vi "HMI Main.vi"() -> ()   [LabVIEW 2014]
panel:
  out "Connected?":bool
  in  "PID Parameters":cluster{"Kp":dbl, "Ki":dbl, "Kd":dbl}
  in  "Set Points":dbl(slide) scale=-10.0..10.0
  in  "RT Target IP":string
  in  "Updata Parameters":bool
  in  "Stop Control":bool
  in  "Start Control":bool
  in  "Connect to Target":bool
  in  "Exit":bool
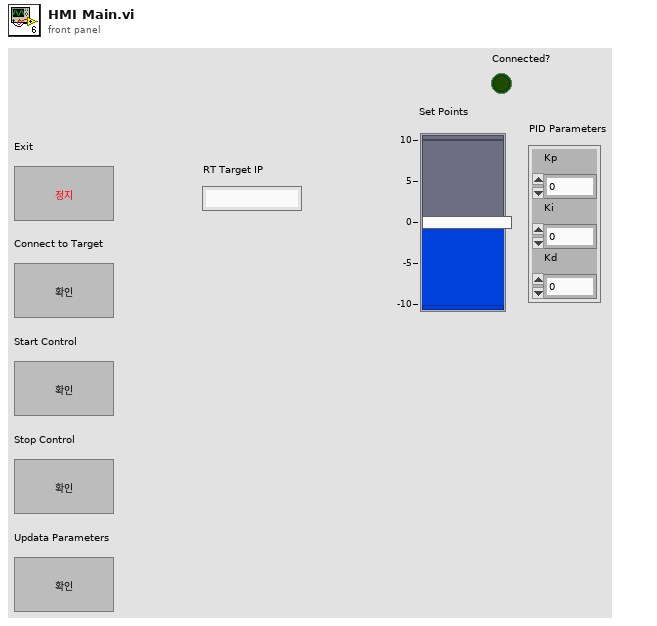
[diagram p1: front panel]
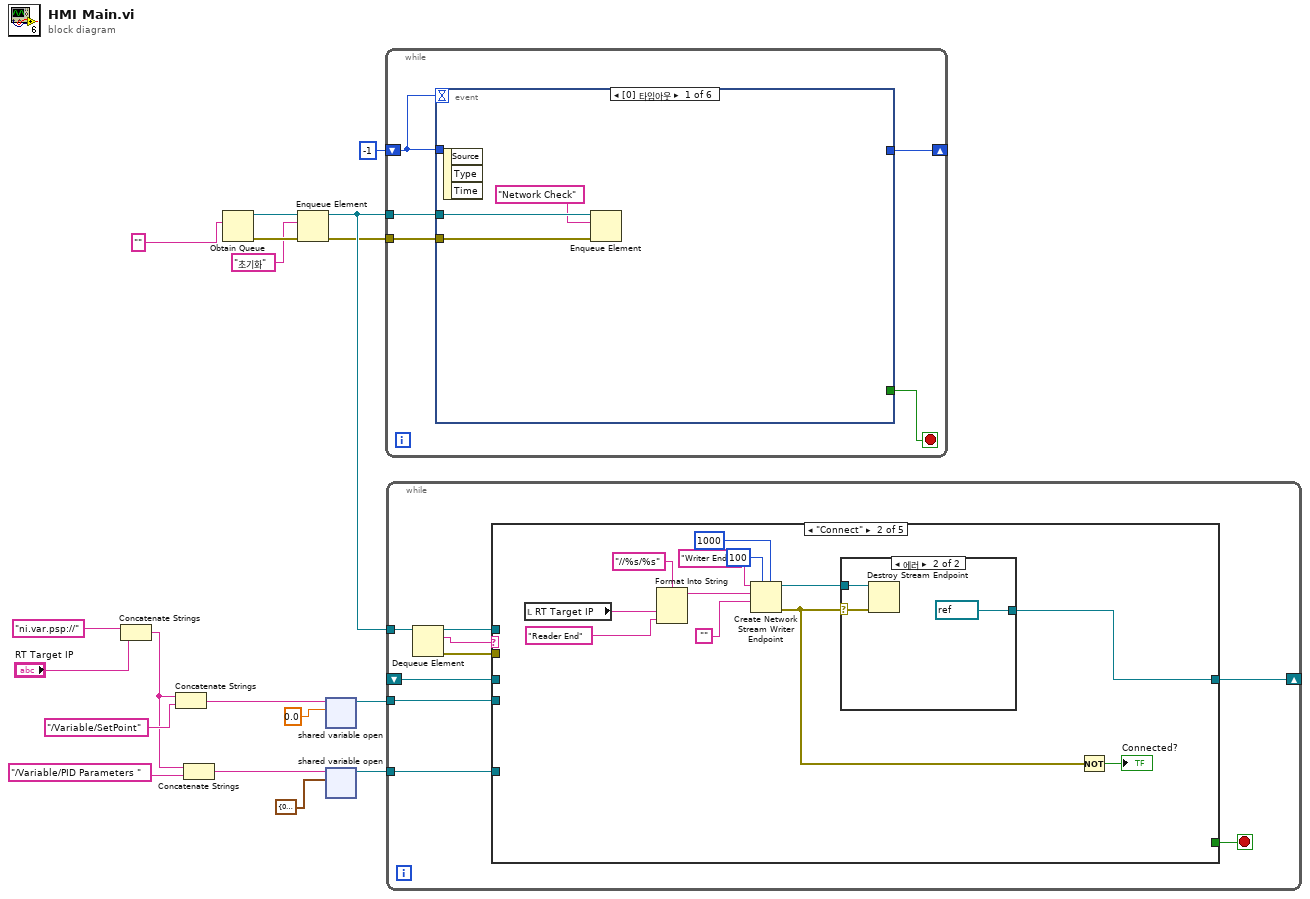
[diagram p0: block diagram]
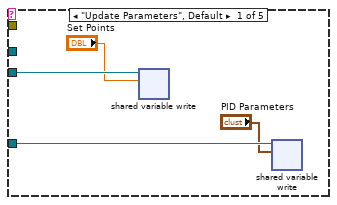
[diagram p2: hidden frame]
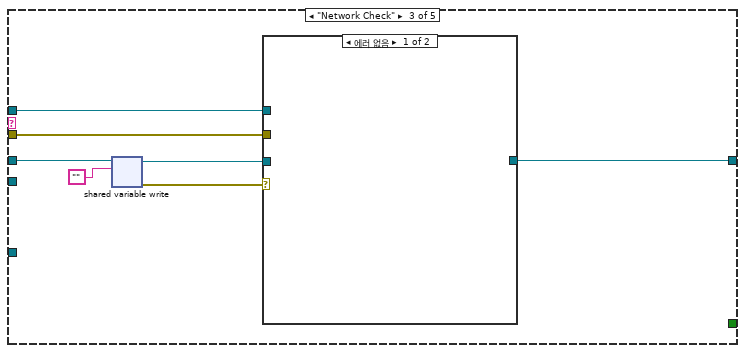
[diagram p4: hidden frame]
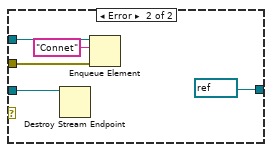
[diagram p5: hidden frame]
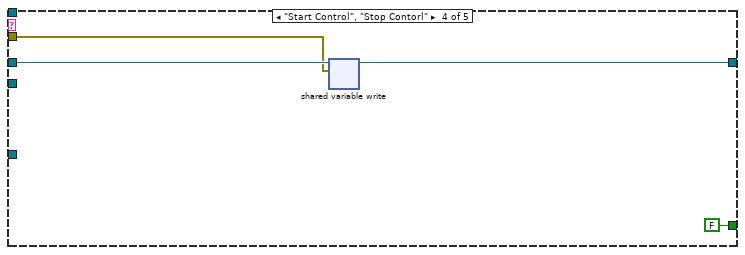
[diagram p6: hidden frame]
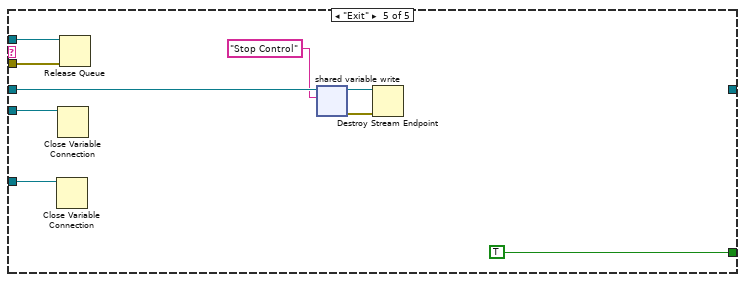
[diagram p7: hidden frame]
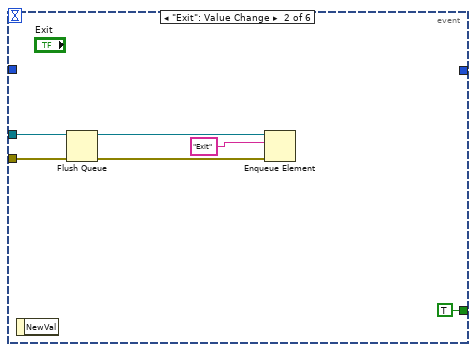
[diagram p8: hidden frame]
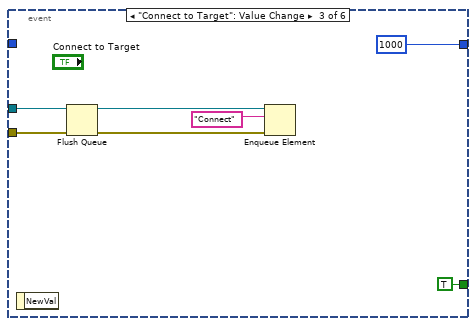
[diagram p9: hidden frame]
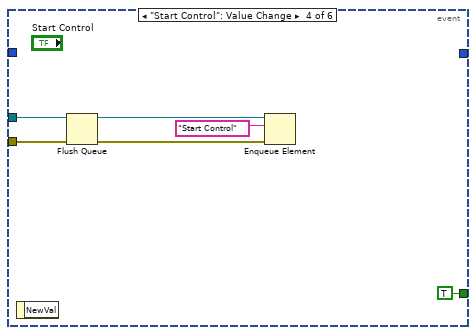
[diagram p10: hidden frame]
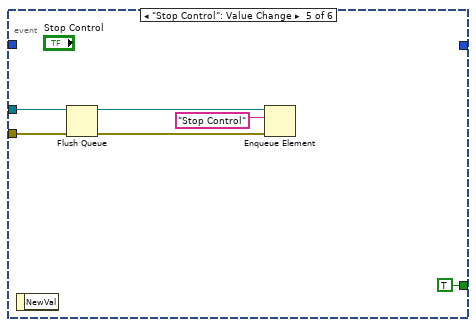
[diagram p11: hidden frame]
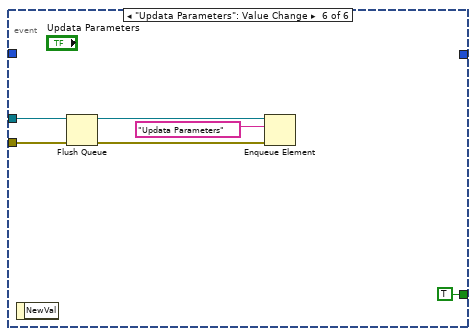
[diagram p12: hidden frame]
diagram:
  n1 = Concatenate Strings("ni.var.psp://", "RT Target IP") -> (w8:string)
  n2 = Concatenate Strings(w8, "/Variable/SetPoint") -> (w6:string)
  n3 = Concatenate Strings(w8, "/Variable/PID Parameters ") -> (w4:string)
  n4 = Obtain Queue(element data type="") -> (queue out=w16:refnum<queue>, error out=w17:errorcluster)  [unwired: 4 in, 1 out]
  n5 = Enqueue Element(queue=w16, element="초기화" ("원소"), error in (no error)=w17) -> (queue out=w15:refnum<queue>, error out=w13:errorcluster)  [unwired: 1 in, 1 out]
  n6 = shared-variable-open(w6, 0.0) -> (w7:refnum<k21>)  [unwired: 2 in, 1 out]
  n7 = shared-variable-open(w4, cluster{"Kp":dbl, "Ki":dbl, "Kd":dbl} {"Kp"=0.0, "Ki"=0.0, "Kd"=0.0} ("PID Parameters")) -> (w5:refnum<k21>)  [unwired: 2 in, 1 out]
  n8 = while {
    tunnel: w15 -> [w23]
    tunnel: w13 -> [w22]
    shift-right: [w20] -> _
    shift-left: -1 -> [w19]
    stop <- w21 stop-if-true
    n9 = event shown="[0] 타임아웃" {
      selector: _ -> [_ _ _ _ _ _]
      dyn-events: _ -> [_ _ _ _ _ _]
      timeout: w19 -> [_ _ _ _ _ _]
      tunnel: w23 -> [w26 w32 w39 w45 w51 w57]
      tunnel: w22 -> [w25 w31 w38 w44 w50 w56]
      tunnel: [_ TRUE TRUE TRUE TRUE TRUE] -> w21
      tunnel: [_ _ 1000 _ _ _] -> w20
      tunnel: w19 -> [_ _ _ _ _ _]
      event Timeout {
        n10 = event-data() -> ()  [unwired: 1 in, 3 out]
        n11 = Enqueue Element(queue=w26, element="Network Check" ("원소"), error in (no error)=w25) -> ()  [unwired: 1 in, 3 out]
      }
      event "Exit": Value Change {
        n12 = event-data() -> ()  [unwired: 1 in, 1 out]
        n13 = Flush Queue(queue=w32, error in (no error)=w31) -> (queue out=w29:refnum<queue>, error out=w28:errorcluster)  [unwired: 1 out]
        n14 = Enqueue Element(queue=w29, element="Exit", error in (no error)=w28) -> ()  [unwired: 1 in, 3 out]
      }
      event "Connect to Target": Value Change {
        n15 = event-data() -> ()  [unwired: 1 in, 1 out]
        n16 = Flush Queue(queue=w39, error in (no error)=w38) -> (queue out=w36:refnum<queue>, error out=w35:errorcluster)  [unwired: 1 out]
        n17 = Enqueue Element(queue=w36, element="Connect", error in (no error)=w35) -> ()  [unwired: 1 in, 3 out]
      }
      event "Start Control": Value Change {
        n18 = event-data() -> ()  [unwired: 1 in, 1 out]
        n19 = Flush Queue(queue=w45, error in (no error)=w44) -> (queue out=w42:refnum<queue>, error out=w41:errorcluster)  [unwired: 1 out]
        n20 = Enqueue Element(queue=w42, element="Start Control", error in (no error)=w41) -> ()  [unwired: 1 in, 3 out]
      }
      event "Stop Control": Value Change {
        n21 = event-data() -> ()  [unwired: 1 in, 1 out]
        n22 = Flush Queue(queue=w51, error in (no error)=w50) -> (queue out=w48:refnum<queue>, error out=w47:errorcluster)  [unwired: 1 out]
        n23 = Enqueue Element(queue=w48, element="Stop Control", error in (no error)=w47) -> ()  [unwired: 1 in, 3 out]
      }
      event "Updata Parameters": Value Change {
        n24 = event-data() -> ()  [unwired: 1 in, 1 out]
        n25 = Flush Queue(queue=w57, error in (no error)=w56) -> (queue out=w54:refnum<queue>, error out=w53:errorcluster)  [unwired: 1 out]
        n26 = Enqueue Element(queue=w54, element="Updata Parameters", error in (no error)=w53) -> ()  [unwired: 1 in, 3 out]
      }
    }
  }
  n27 = while {
    tunnel: w15 -> [w66]
    tunnel: w7 -> [w61]
    tunnel: w5 -> [w60]
    shift-right: [w59] -> _
    shift-left: _ -> [w58]
    stop <- w62 stop-if-true
    n28 = Dequeue Element(queue=w66) -> (queue out=w64:refnum<queue>, element=w65:string, error out=w63:errorcluster)  [unwired: 2 in, 1 out]
    n29 = case shown="\"Connect\"" w65 {
      tunnel: w64 -> [_ _ w89 _ w110]
      tunnel: w63 -> [_ _ w88 w98 w109]
      tunnel: [_ _ _ FALSE TRUE] -> w62
      tunnel: w61 -> [w70 _ _ _ w106]
      tunnel: w60 -> [w69 _ _ _ w107]
      tunnel: [_ w74 w86 w100 _] -> w59
      tunnel: w58 -> [_ _ w92 w101 w105]
      frame "Update Parameters", Default {
        n30 = shared-variable-write(w70, "Set Points") -> ()  [unwired: 1 in, 2 out]
        n31 = shared-variable-write(w69, "PID Parameters") -> ()  [unwired: 1 in, 2 out]
      }
      frame "Connect" {
        n32 = local read "RT Target IP"() -> (w82:string)
        n33 = Format Into String(format string="//%s/%s" ("포맷 문자열"), w82, "Reader End" ("입력 2")) -> (resulting string=w79:string)  [unwired: 2 in, 1 out]
        n34 = Create Network Stream Writer Endpoint(5:1000 ("타임아웃(ms) (-1)"), 7:100 ("발신자 버퍼 크기"), 9:"", 10:w79, 11:"Writer End" ("발신자 이름")) -> (0:w77:errorcluster, 3:w78:refnum<k21>)  [unwired: 2 in]
        n35 = case shown="에러" w77 {
          selector: w77 -> [_ w85]
          tunnel: w78 -> [_ w84]
          tunnel: [_ refnum<k21> refnum ("발신자 이름")] -> w74
          frame No Error {
          }
          frame Error {
            n36 = Destroy Stream Endpoint(8:w85, 11:w84) -> ()  [unwired: 1 out]
          }
        }
        n37 = Not(x=w77) -> (.not. x?=→"Connected?":bool)
      }
      frame "Network Check" {
        n38 = shared-variable-write(w92, "") -> (w87:refnum<k21>, w90:errorcluster)  [unwired: 2 in, 1 out]
        n39 = case shown="에러 없음" w90 {
          tunnel: w89 -> [_ w97]
          tunnel: w88 -> [_ w95]
          tunnel: w87 -> [_ w94]
          tunnel: [_ refnum<k21> refnum ("발신자 이름")] -> w86
          frame No Error {
          }
          frame Error {
            n40 = Destroy Stream Endpoint(11:w94) -> ()  [unwired: 1 in, 1 out]
            n41 = Enqueue Element(queue=w97, element="Connet" ("원소"), error in (no error)=w95) -> ()  [unwired: 1 in, 3 out]
          }
        }
      }
      frame "Start Control", "Stop Contorl" {
        n42 = shared-variable-write(w101, w98) -> (w100:refnum<k21>)  [unwired: 2 in, 2 out]
      }
      frame "Exit" {
        n43 = Close Variable Connection(11:w107) -> ()  [unwired: 1 in, 1 out]
        n44 = Close Variable Connection(11:w106) -> ()  [unwired: 1 in, 1 out]
        n45 = Release Queue(queue=w110, error in (no error)=w109) -> ()  [unwired: 1 in, 3 out]
        n46 = shared-variable-write(w105, "Stop Control") -> (w103:refnum<k21>, w104:errorcluster)  [unwired: 2 in, 1 out]
        n47 = Destroy Stream Endpoint(8:w104, 11:w103) -> ()  [unwired: 1 out]
      }
    }
  }
